vi "dump_comment.vi"(10 "left pad (\"\")":string, 11 "comment in":string) -> (3 "comment out":string)   [LabVIEW 2017, in "rpacini_toml.lvlib"]
uses:
  rpacini_toml.lvlib
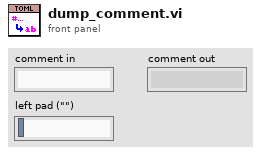
[diagram p1: front panel]
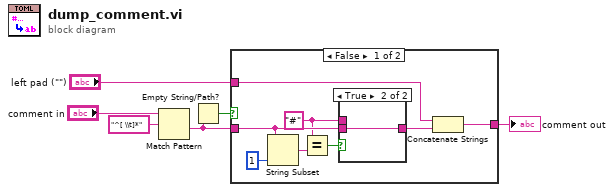
[diagram p0: block diagram]
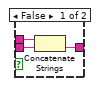
[diagram p2: hidden frame]
diagram:
  n1 = Match Pattern(string="comment in", regular expression="^[ \\t]*") -> (after substring=w2:string)  [unwired: 1 in, 3 out]
  n2 = Empty String/Path?(string/path=w2) -> (empty?=w5:bool)
  n3 = case shown="False" w5 {
    tunnel: [w8 _] -> w6
    tunnel: w2 -> [w12 _]
    tunnel: "left pad (\"\")" -> [w7 _]
    frame False {
      w11 = "#" ("y")
      n4 = String Subset(string=w12, length (rest)=1 ("length (rest)")) -> (substring=w13:string)  [unwired: 1 in]
      n5 = Equal?(x=w11, y=w13) -> (x = y?=w9:bool)
      n6 = case shown="True" w9 {
        tunnel: w12 -> [w17 w18]
        tunnel: w11 -> [w16 _]
        tunnel: [w15 w18] -> w10
        frame False {
          n7 = Concatenate Strings(w16, w17) -> (w15:string)
        }
        frame True {
        }
      }
      n8 = Concatenate Strings(w7, w10) -> (w8:string)
    }
    frame True {
    }
  }
  "comment out" <- w6
